vi "俄罗斯方块-存储形状数组.vi"(6 "Y":i8, 7 "X":i8, 8 "当前形状数组":u32[][](array[numeric]), 9 "主窗数组输入":u32[][](array[numeric])) -> (3 "主窗数组输出":u32[][](array[numeric]))   [LabVIEW 2016]
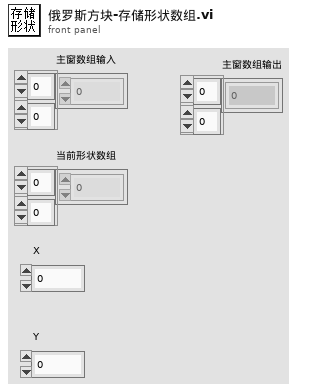
[diagram p1: front panel]
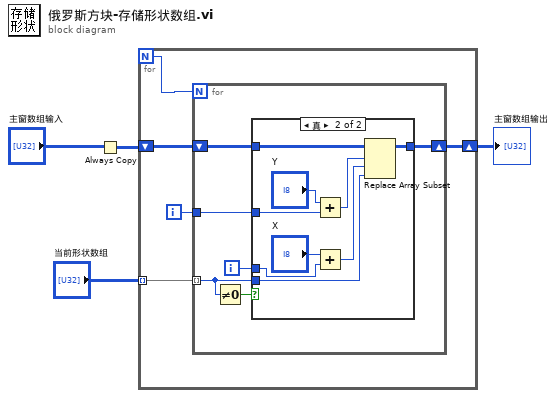
[diagram p0: block diagram]
diagram:
  n1 = Always Copy(1:"主窗数组输入") -> (0:w2:u32[][])
  n2 = for {
    N -> [w9]
    tunnel: "当前形状数组" -> [w8] mode=indexing
    shift-right: [w6] -> w4
    shift-left: w2 -> [w7]
    i -> [w5]
    n3 = for {
      N: w9 -> [_]
      tunnel: w8 -> [w13] mode=indexing
      shift-right: [w12] -> w6
      shift-left: w7 -> [w14]
      tunnel: w5 -> [w11]
      i -> [w10]
      n4 = Not Equal To 0?(x=w13) -> (x != 0?=w15:bool)
      n5 = case shown="真" w15 {
        tunnel: w14 -> [w16 w25]
        tunnel: w13 -> [_ w24]
        tunnel: [w16 w23] -> w12
        tunnel: w11 -> [_ w21]
        tunnel: w10 -> [_ w20]
        frame False {
        }
        frame True {
          n6 = Add(x="Y", y=w21) -> (x+y=w22:i32)
          n7 = Add(x="X", y=w20) -> (x+y=w19:i32)
          n8 = Replace Array Subset(array=w25, new element=w24, index (row)=w22, index (col)=w19) -> (w23:u32[][])
        }
      }
    }
  }
  "主窗数组输出" <- w4
